vi "PhotonCamera_IsConnected.vi"(8 "Pass_Through_Time":dbl=-1.0 format="%33.4f", 11 "CameraName":string) -> (3 "IsConnected":bool)   [LabVIEW 2019, in "PhotonVisionLib.lvlib"]
doc: "Determines if communications to camera is valid.\n\nInputs:\n - CameraName -- The nickname of the camera (found in the PhotonVision UI).\n \nOutputs:\n - IsConnected -- TRUE if communications have been received within the last 0.5 seconds."
uses:
  PhotonVisionLib.lvlib
  <vilib>/Rock Robotics/Network Tables/NT Read Number.vi
  <vilib>/Rock Robotics/WPI/ThirdParty/JAS_Junk/TrajLib/Trajectory_Library.lvlib
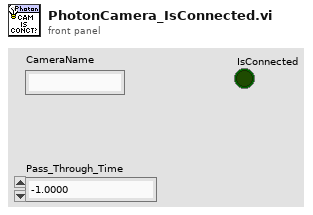
[diagram p1: front panel]
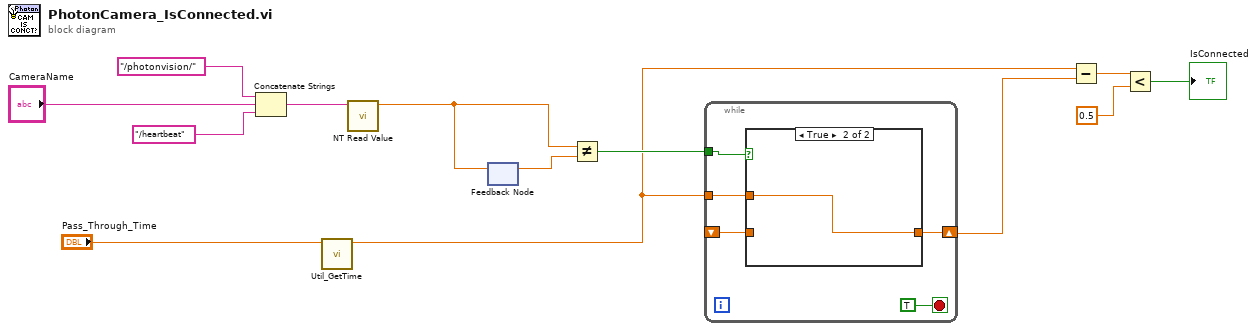
[diagram p0: block diagram]
diagram:
  n1 = Concatenate Strings("/photonvision/", "CameraName", "/heartbeat") -> (w10:string)
  n2 = call <vilib>:"Util_GetTime.vi"("Pass_Through_Time"="Pass_Through_Time") -> ("FPGA_Time_Seconds"=w5:dbl)  [unwired: 8 in, 2 out]
  n3 = call-poly <vilib>:"NT Read Value.vi"("Name"=w10) -> ("Numeric"=w6:dbl)  [unwired: 9 in, 1 out]
  n4 = feedback-in #1(w6) -> ()
  n5 = feedback #1() -> (w8:dbl)  [unwired: 1 in]
  n6 = Not Equal?(x=w6, y=w8) -> (x != y?=w7:bool)
  n7 = while {
    tunnel: w7 -> [w17]
    tunnel: w5 -> [w16]
    shift-right: [w15] -> w4
    shift-left: _ -> [w14]
    stop <- TRUE stop-if-true
    n8 = case shown="True" w17 {
      tunnel: [w19 w20] -> w15
      tunnel: w16 -> [_ w20]
      tunnel: w14 -> [w19 _]
      frame False {
      }
      frame True {
      }
    }
  }
  n9 = Subtract(x=w5, y=w4) -> (x-y=w3:dbl)
  n10 = Less?(x=w3, y=0.5) -> (x < y?=→"IsConnected":bool)
